vi "Wait for Acquisition Complete.vi"(8 "error in (no error)":errorcluster, 9 "Maximum Time (10000)":u32=10000, 11 "VISA resource name":refnum<visa-resource-name>) -> (0 "error out":errorcluster, 3 "VISA resource name out":refnum<visa-resource-name>)   [LabVIEW 2021, in "Ceyear.lvlib"]
doc: "Waits for the current sweep to finish. This VI should be called after <b>Initiate</b> VI and before <b>Fetch Trace</b> VI.\n\n<B>Note:</B> \n\nUse this VI only with other low-level VIs. The high-level VIs automatically incorporate this functionality. This VI does not check the instrument status."
uses:
  <instrlib>/Ceyear/Ceyear.lvlib
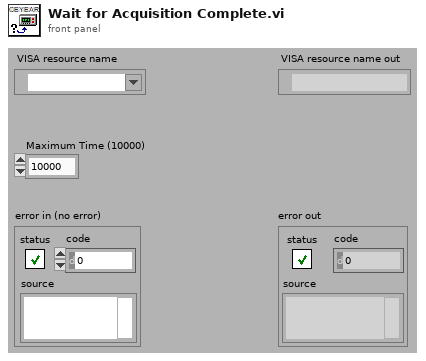
[diagram p1: front panel]
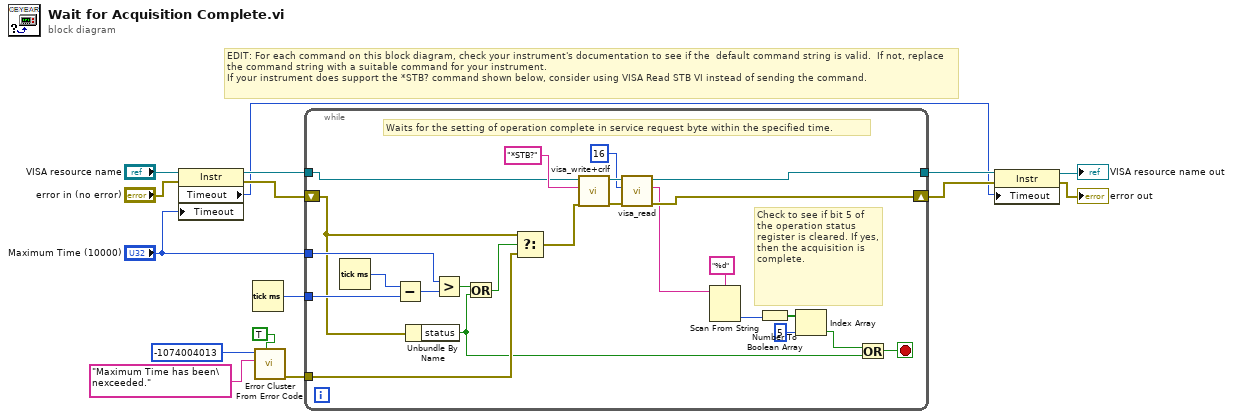
[diagram p0: block diagram]
diagram:
  # "EDIT: For each command on this block diagram, check your instrument's documentation to see if the  default command string is valid.  If not, replace the command string with a suitable command for your instrument. \nIf your instrument does support the *STB? command shown below, consider using VISA Read STB VI instead of sending the command."
  n1 = property class="Instr"(reference="VISA resource name", error in="error in (no error)", "Timeout"="Maximum Time (10000)") -> (reference out=w3:refnum<visa-resource-name>, error out=w2:errorcluster, "Timeout"=w1:u32)
  n2 = Tick Count (ms)() -> (millisecond timer value=w15:u32)
  n3 = call <vilib>:"Error Cluster From Error Code.vi"("show call chain? (False)"=TRUE, "error message (\"\")"="Maximum Time has been\nexceeded." ("error message (\"\")"), "error code (0)"=-1074004013) -> ("error out"=w11:errorcluster)  [unwired: 6 in]
  n4 = while {
    tunnel: [w18] -> w9
    tunnel: w3 -> [w20]
    tunnel: "Maximum Time (10000)" -> [w35]
    tunnel: w15 -> [w36]
    shift-right: [w17] -> w10
    shift-left: w2 -> [w28]
    tunnel: w11 -> [w27]
    stop <- w31 stop-if-true
    # "Waits for the setting of operation complete in service request byte within the specified time."
    # "Check to see if bit 5 of the operation status register is cleared. If yes, then the acquisition is complete."
    n5 = Tick Count (ms)() -> (millisecond timer value=w38:u32)
    n6 = Subtract(x=w38, y=w36) -> (x-y=w37:u32)
    n7 = Unbundle By Name(w28) -> ("status"=w25:bool)
    n8 = Greater?(x=w35, y=w37) -> (0:w26:bool)
    n9 = Or(x=w26, y=w25) -> (x .or. y?=w29:bool)
    n10 = Select(t=w28, s=w29, f=w27) -> (s? t:f=w19:errorcluster)
    n11 = call <instrlib>:"visa_write+crlf.vi"("error in (no error)"=w19, "Strings (empty)"="*STB?" ("write buffer"), "VISA resource name"=w20) -> ("error out"=w24:errorcluster, "VISA resource name out"=w23:refnum<visa-resource-name>)  [unwired: 7 in]
    n12 = call <instrlib>:"visa_read.vi"("error in (no error)"=w24, "Byte Count (0)"=u32 16 ("byte count"), "VISA resource name"=w23) -> ("error out"=w17:errorcluster, "Read Data"=w16:string, "VISA resource name out"=w18:refnum<visa-resource-name>)  [unwired: 5 in, 1 out]
    n13 = Scan From String(format string="%d", input string=w16) -> (output 1=w33:i32)  [unwired: 3 in, 3 out]
    n14 = Number To Boolean Array(number=w33) -> (Boolean array=w32:bool[])
    n15 = Index Array(array=w32, index=5) -> (element=w30:bool)
    n16 = Or(x=w30, y=w25) -> (x .or. y?=w31:bool)
  }
  n17 = property class="Instr"(reference=w9, error in=w10, "Timeout"=w1) -> (reference out=→"VISA resource name out":refnum<visa-resource-name>, error out=→"error out":errorcluster)
